vi "Initialize Pointers.vi"(8 "error in (no error)":errorcluster, 10 "framework configuration":T1, 11 "VeriStand DSF in":refnum<class "VeriStand DSF.lvclass">) -> (0 "error out":errorcluster, 3 "VeriStand DSF out":refnum<class "VeriStand DSF.lvclass">)   [LabVIEW 2017, in "DSF Engine.lvlib" / "VeriStand DSF.lvclass"]
uses:
  VeriStand DSF.lvclass
  DSF Core.lvlibp/Classes/Configuration/Configuration Session.lvclass
  DSF Core.lvlibp/Classes/Configuration/Channel Count (Transfer).vi
  DSF Core.lvlibp/Classes/Configuration/Transfer Count (Transfer Group).vi
  DSF Core.lvlibp/Classes/Configuration/Transfer Group Count (Plugin).vi
  DSF Core.lvlibp/Classes/Configuration/Largest Buffer Size (Transfer Group).vi
  DSF Core.lvlibp/Classes/Configuration/Required Buffer Size (Transfer).vi
  DSF Core.lvlibp/Classes/Configuration/Transfer Group Count (Framework).vi
  DSF Core.lvlibp/Typedefs/DSF Timing Info.ctl
  DSF Core.lvlibp
  DSF Core.lvlibp/Typedefs/DSF Settings Info.ctl
  DSF Core.lvlibp/Typedefs/DSF Engine Plugin Thread Configuration.ctl
  DSF Core.lvlibp/Typedefs/DSF Direction.ctl
  DSF Core.lvlibp/Typedefs/DSF Byte Order.ctl
  DSF Core.lvlibp/Typedefs/DSF Data Type.ctl
  DSF Core.lvlibp/Typedefs/DSF Engine Channel Configuration.ctl
  DSF Core.lvlibp/Typedefs/DSF Engine Transfer Configuration.ctl
  DSF Core.lvlibp/Typedefs/DSF Timeout Behavior.ctl
  DSF Core.lvlibp/Typedefs/DSF Engine Transfer Group Configuration.ctl
  DSF Core.lvlibp/Typedefs/DSF Engine Plugin Configuration.ctl
  DSF Core.lvlibp/Typedefs/DSF Engine Framework Configuration.ctl
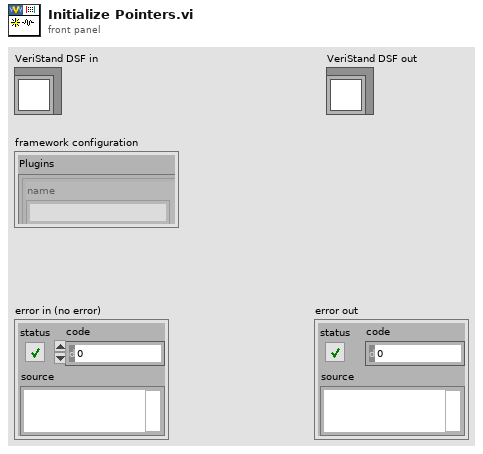
[diagram p1: front panel]
types:
  T1 = typedef "DSF Core.lvlibp/DSF Engine Framework Configuration.ctl" = cluster{"Plugins":T2[]}
  T2 = typedef "DSF Core.lvlibp/DSF Engine Plugin Configuration.ctl" = cluster{"name":string, "components":string[], "cycle timing":T3, "threads":T4[], "Transfer Groups":T6[], "settings":T5}
  T3 = typedef "DSF Core.lvlibp/DSF Timing Info.ctl" = cluster{"priority":u64, "decimation":u64, "offset":u64}
  T4 = typedef "DSF Core.lvlibp/DSF Engine Plugin Thread Configuration.ctl" = cluster{"buffer converter settings":T5, "transceiver settings":T5, "custom settings":T5, "processor":i32, "priority offset":i16}
  T5 = typedef "DSF Core.lvlibp/DSF Settings Info.ctl" = cluster{"key":string, "value":string}[]
  T6 = typedef "DSF Core.lvlibp/DSF Engine Transfer Group Configuration.ctl" = cluster{"name":string, "direction":T7, "cycle timing":T3, "thread index":i32, "settings":T5, "Transfers":T8[], "timeout behavior":T12}
  T7 = typedef "DSF Core.lvlibp/DSF Direction.ctl" = enum8{"Tx", "Rx"}
  T8 = typedef "DSF Core.lvlibp/DSF Engine Transfer Configuration.ctl" = cluster{"name":string, "byte order":T9, "settings":T5, "channels":T10[]}
  T9 = typedef "DSF Core.lvlibp/DSF Byte Order.ctl" = enum8{"big-endian", "little-endian"}
  T10 = typedef "DSF Core.lvlibp/DSF Engine Channel Configuration.ctl" = cluster{"string offset":u64, "string data type":T11, "engine data type":T11, "name":string, "settings":T5, "units":string}
  T11 = typedef "DSF Core.lvlibp/DSF Data Type.ctl" = enum8{"Bool", "SGL", "DBL", "I8", "I16", "I32", "I64", "U8", "U16", "U32", "U64"}
  T12 = typedef "DSF Core.lvlibp/DSF Timeout Behavior.ctl" = enum8{"Increment Late Count", "Throw Error"}
  T13 = enum16{"open", "replace", "create", "open or create", "replace or create", "replace or create with confirmation"}
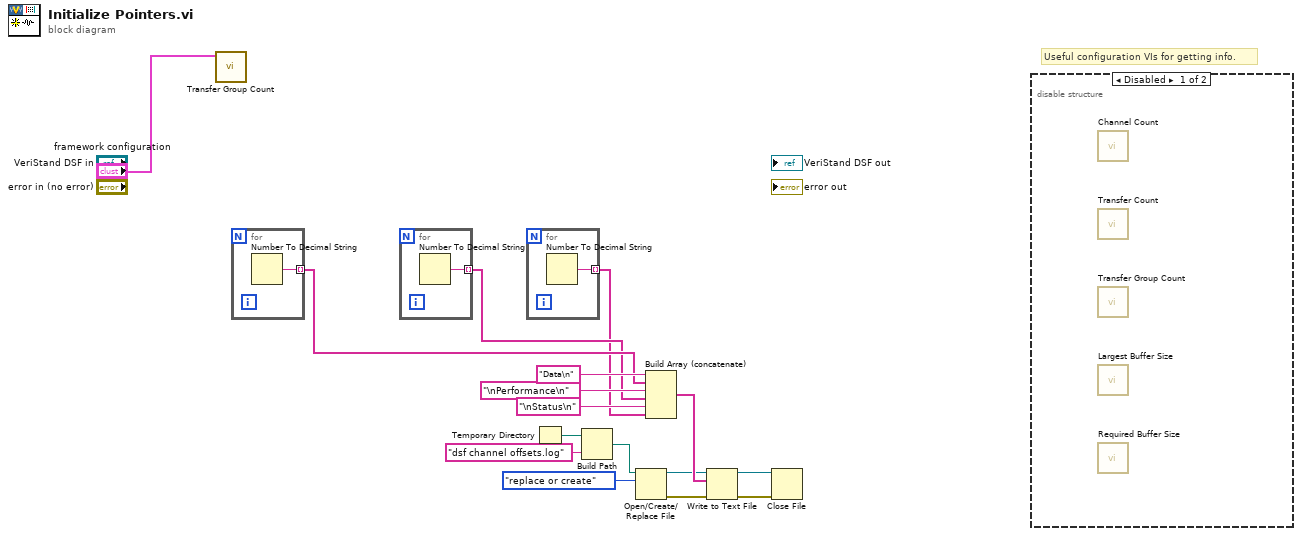
[diagram p0: block diagram]
diagram:
  # "Useful configuration VIs for getting info."
  n1 = call-poly "Transfer Group Count.vi"("Framework Configuration in"="framework configuration") -> ()  [unwired: 8 in, 3 out]
  n2 = for {
    tunnel: [w17] -> w4 mode=indexing
    n3 = Number To Decimal String() -> (decimal integer string=w17:string)  [unwired: 2 in]
  }
  n4 = for {
    tunnel: [w18] -> w3 mode=indexing
    n5 = Number To Decimal String() -> (decimal integer string=w18:string)  [unwired: 2 in]
  }
  n6 = for {
    tunnel: [w19] -> w2 mode=indexing
    n7 = Number To Decimal String() -> (decimal integer string=w19:string)  [unwired: 2 in]
  }
  n8 = Temporary Directory() -> (w6:path)
  n9 = Build Path(base path=w6, name or relative path="dsf channel offsets.log") -> (appended path=w8:path)
  n10 = Open/Create/Replace File(file path (use dialog)=w8, operation (0:open)=T13."replace or create") -> (refnum out=w9:refnum<file>, error out=w10:errorcluster)  [unwired: 4 in, 1 out]
  n11 = Build Array (concatenate)("Data\n", w4, "\nPerformance\n", w3, "\nStatus\n", w2) -> (w16:string[])
  n12 = Write to Text File(file (use dialog)=w9, text=w16, error in=w10) -> (refnum out=w12:refnum<file>, error out=w11:errorcluster)  [unwired: 1 in, 1 out]
  n13 = Close File(refnum=w12, error in=w11) -> ()  [unwired: 2 out]
  n14 = disable-structure shown="Disabled" {
    frame Disabled {
      n15 = call-poly "Channel Count.vi"() -> ()  [unwired: 9 in, 3 out]
      n16 = call-poly "Transfer Count.vi"() -> ()  [unwired: 9 in, 3 out]
      n17 = call-poly "Transfer Group Count.vi"() -> ()  [unwired: 9 in, 3 out]
      n18 = call-poly "Largest Buffer Size.vi"() -> ()  [unwired: 8 in, 4 out]
      n19 = call-poly "Required Buffer Size.vi"() -> ()  [unwired: 8 in, 4 out]
    }
    frame Enabled {
    }
  }
